vi "素材.vi"() -> ()   [LabVIEW 2018]
uses:
  <vilib>/Analysis/4window.llb/windowTd.ctl
  <vilib>/measure/maspectr.llb/FFT Spectrum (Mag-Phase) for 1 Chan.vi
  <vilib>/measure/macond.llb/IIR Filter for 1 Chan.vi
  <vilib>/measure/NI_MABase.lvlib
  <vilib>/measure/NI_MAPro.lvlib
  <vilib>/Analysis/NI_AALPro.lvlib
panel:
  out "波形图 2":dbl[](graph)
  out "波形图":cluster{"f0":dbl, "df":dbl, dbl[]}[](graph)
  in  "window":T1=1 caption="窗" items=["矩形"=0, "Hanning"=1, "Hamming"=2, "Blackman-Harris"=3, "Exact Blackman"=4, "Blackman"=5, "Flat Top"=6, "4阶Blackman-Harris "=7, "7阶Blackman-Harris"=8, "Low Sidelobe"=9, "Blackman Nuttall"=11, "三角"=30, "Bartlett-Hanning"=31, "Bohman"=32, "Parzen"=33, "Welch"=34, "Kaiser"=60, "Dolph-Chebyshev"=61, "高斯"=62]
  in  "IIR filter specifications":T2={"Topology"=enum."Butterworth", "Type"=enum."Lowpass", "Order"=1, "Lower Fc"=100.0, "Upper Fc"=200.0, "PB Ripple"=1.0, "SB Attenuation"=60.0} caption="IIR滤波器规范" {"PB Ripple" format="%0.2f"; "SB Attenuation" format="%0.2f"; "Lower Fc" format="%0.2p"; "Upper Fc" format="%0.2p"}
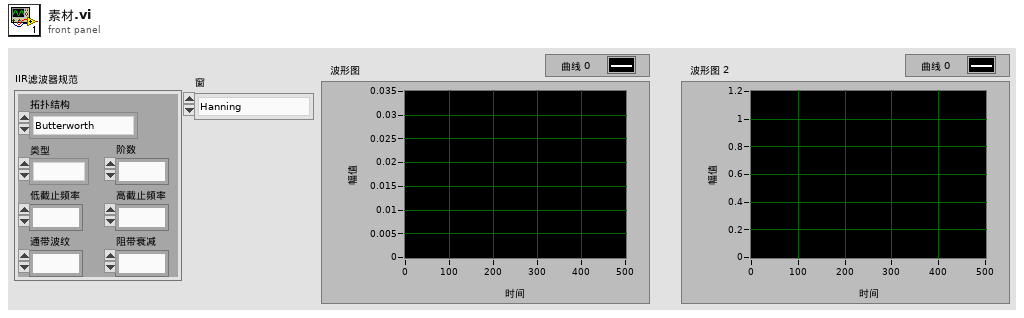
[diagram p1: front panel]
types:
  T1 = typedef "NI_AALPro.lvlib/windowTd.ctl" = u32
  T2 = cluster{"Topology":enum16{"Off", "Butterworth", "Chebyshev", "Inverse Chebyshev", "Elliptic", "Bessel"}, "Type":enum16{"Lowpass", "Highpass", "Bandpass", "Bandstop"}, "Order":i32, "Lower Fc":dbl, "Upper Fc":dbl, "PB Ripple":dbl, "SB Attenuation":dbl}
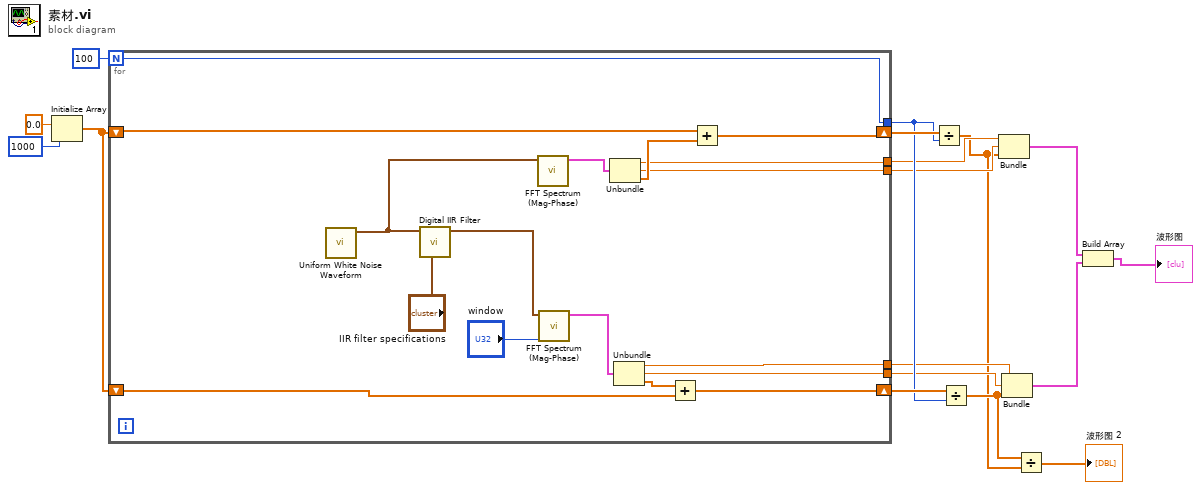
[diagram p0: block diagram]
diagram:
  n1 = Initialize Array(0.0 ("元素"), 1000 ("维数大小")) -> (w13:dbl[])
  n2 = for {
    N: 100 -> [w26]
    shift-right: [w28] -> w14
    shift-left: w13 -> [w27]
    tunnel: [w26] -> w11
    shift-right: [w23] -> w12
    shift-left: w13 -> [w22]
    tunnel: [w21] -> w10
    tunnel: [w20] -> w9
    tunnel: [w19] -> w8
    tunnel: [w18] -> w7
    n3 = call <vilib>:"Uniform White Noise Waveform.vi"() -> ("signal out"=w31:waveform(dbl))  [unwired: 10 in, 1 out]
    n4 = call-poly <vilib>:"Digital IIR Filter.vi"("IIR filter specifications"="IIR filter specifications", "signal in"=w31) -> ("signal out"=w33:waveform(dbl))  [unwired: 7 in, 2 out]
    n5 = call-poly <vilib>:"FFT Spectrum (Mag-Phase).vi"("time signal"=w31) -> ("magnitude"=w30:cluster{"f0":dbl, "df":dbl, "magnitude":dbl[]})  [unwired: 6 in, 4 out]
    n6 = call-poly <vilib>:"FFT Spectrum (Mag-Phase).vi"("window"="window", "time signal"=w33) -> ("magnitude"=w25:cluster{"f0":dbl, "df":dbl, "magnitude":dbl[]})  [unwired: 5 in, 4 out]
    n7 = Unbundle(w30) -> ("f0"=w21:dbl, "df"=w20:dbl, "magnitude"=w29:dbl[])
    n8 = Unbundle(w25) -> ("f0"=w18:dbl, "df"=w19:dbl, "magnitude"=w24:dbl[])
    n9 = Add(x=w24, y=w22) -> (x+y=w23:dbl[])
    n10 = Add(x=w27, y=w29) -> (x+y=w28:dbl[])
  }
  n11 = Divide(x=w14, y=w11) -> (x/y=w2:dbl[])
  n12 = Divide(x=w12, y=w11) -> (x/y=w3:dbl[])
  n13 = Bundle("f0"=w10, "df"=w9, w2) -> (w6:cluster{"f0":dbl, "df":dbl, dbl[]})  [unwired: 1 in]
  n14 = Bundle("f0"=w7, "df"=w8, w3) -> (w5:cluster{"f0":dbl, "df":dbl, dbl[]})  [unwired: 1 in]
  n15 = Divide(x=w3, y=w2) -> (x/y=→"波形图 2":dbl[])
  n16 = Build Array(w6, w5) -> (→"波形图":cluster{"f0":dbl, "df":dbl, dbl[]}[])
